vi "课堂.vi"() -> ()   [LabVIEW 2025]
uses:
  <vilib>/Utility/file.llb/Write Delimited Spreadsheet (DBL).vi
  <vilib>/Utility/file.llb/Read Delimited Spreadsheet (DBL).vi
panel:
  out "状态显示 2":string
  out "温度计 2":dbl(slide) scale=0.0..100.0
  out "报警显示 2":bool
  in  "温度下限 2":dbl=10.0
  in  "温度上限 2":dbl=50.0
  out "温度计":dbl(slide) scale=0.0..100.0
  out "报警显示":bool
  out "状态显示":string
  in  "温度下限":dbl=10.0
  in  "温度上限":dbl=50.0
  out "布尔":bool
  in  "滑动杆":dbl(slide) scale=0.0..10.0
  in  "文本 3":string="NIHAO"
  in  "操作(0:open) 3":T1(ring)
  in  "文件路径（使用对话框） 3":path
  in  "数值 3":i32=10
  out "文本 2":string
  in  "操作(0:open) 2":T1(ring)
  in  "文件路径（使用对话框） 2":path
  in  "文本":string
  in  "数值 2":i32=10
  in  "操作(0:open)":T1(ring)
  in  "文件路径（使用对话框）":path
  out "all rows":dbl[][](array[numeric]) caption="所有行"
  in  "number of rows (all:-1)":i32=-1 caption="行数（全部:-1）"
  out "new file path (Not A Path if cancelled) 2":path caption="新建文件路径（取消时为非法路径）"
  in  "file path (dialog if empty) 2":path caption="文件路径（空时为对话框）"
  in  "transpose? (no:F)":bool caption="转置（否:F）"
  in  "format (%.3f)":string="%.3f" caption="格式(%.3f)"
  in  "delimiter (\\t)":string="\t" caption="分隔符(\\t)"
  in  "append to file? (new file:F)":bool caption="添加至文件？（新文件：F）"
  in  "数值":i32=10
  in  "file path (dialog if empty)":path caption="文件路径（空时为对话框）"
  out "new file path (Not A Path if cancelled)":path caption="新建文件路径（取消时为非法路径）"
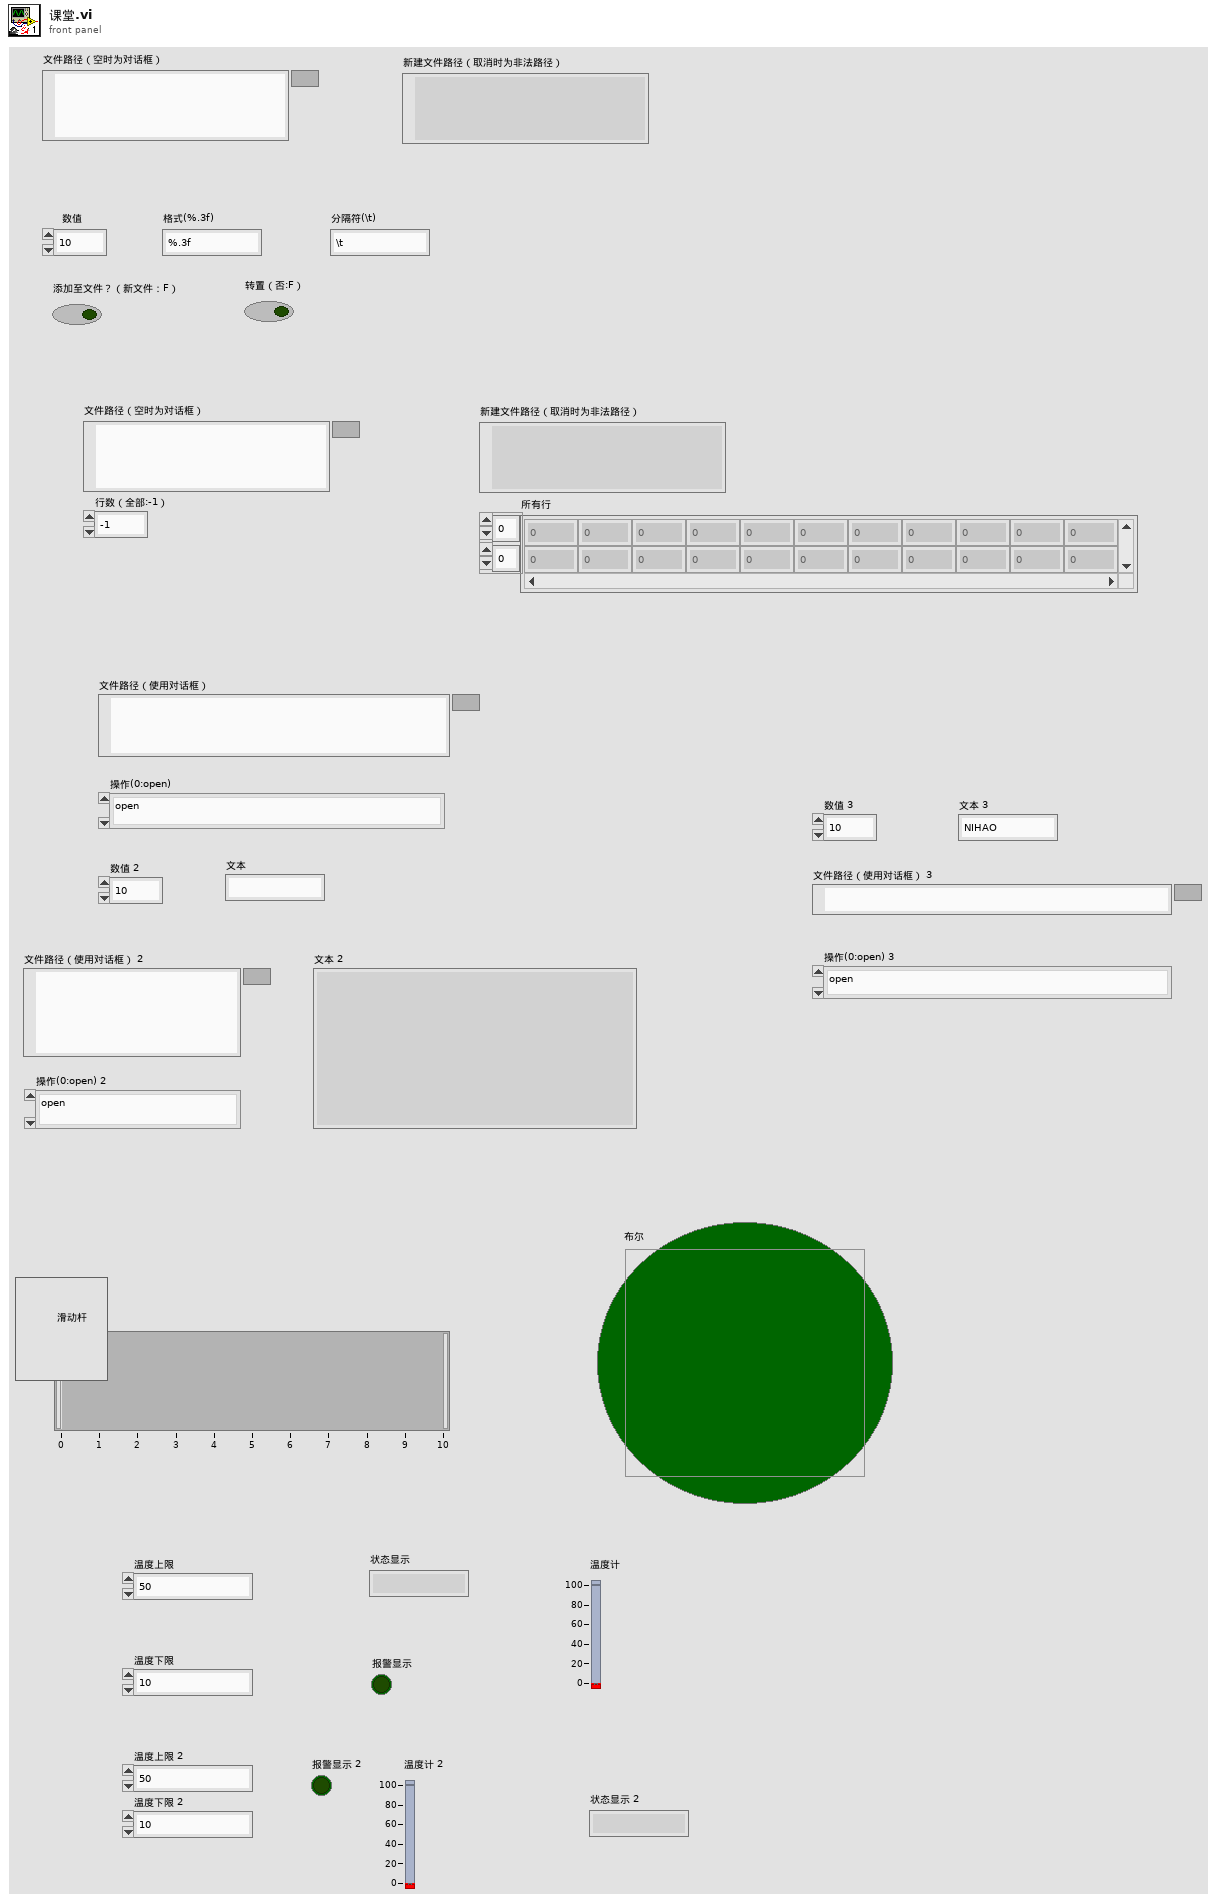
[diagram p1: front panel]
types:
  T1 = enum16{"open", "replace", "create", "open or create", "replace or create", "replace or create with confirmation"}
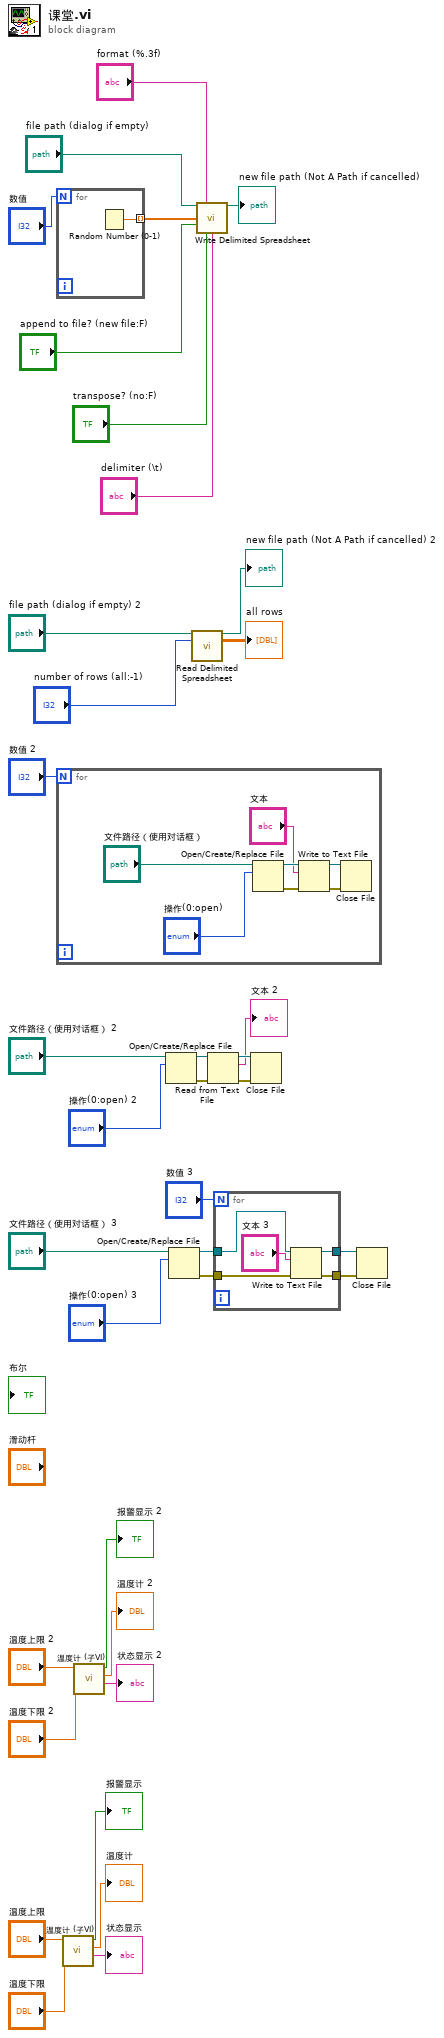
[diagram p0: block diagram]
diagram:
  n1 = for {
    N: "数值" -> [_]
    tunnel: [w38] -> w34 mode=indexing
    n2 = Random Number (0-1)() -> (number: 0 to 1=w38:dbl)
  }
  n3 = for {
    N: "数值 2" -> [_]
    n4 = Open/Create/Replace File(file path (use dialog)="文件路径（使用对话框）", operation (0:open)="操作(0:open)") -> (refnum out=w44:refnum<file>, error out=w40:errorcluster)  [unwired: 4 in, 1 out]
    n5 = Write to Text File(file (use dialog)=w44, text="文本", error in=w40) -> (refnum out=w41:refnum<file>, error out=w39:errorcluster)  [unwired: 1 in, 1 out]
    n6 = Close File(refnum=w41, error in=w39) -> ()  [unwired: 2 out]
  }
  n7 = call "温度计 (子VI).vi"("温度下限"="温度下限", "温度上限"="温度上限") -> ("状态显示"=→"状态显示":string, "温度计"=→"温度计":dbl, "报警显示"=→"报警显示":bool)  [unwired: 7 in]
  n8 = call "温度计 (子VI).vi"("温度下限"="温度下限 2", "温度上限"="温度上限 2") -> ("状态显示"=→"状态显示 2":string, "温度计"=→"温度计 2":dbl, "报警显示"=→"报警显示 2":bool)  [unwired: 7 in]
  n9 = Open/Create/Replace File(file path (use dialog)="文件路径（使用对话框） 2", operation (0:open)="操作(0:open) 2") -> (refnum out=w22:refnum<file>, error out=w19:errorcluster)  [unwired: 4 in, 1 out]
  n10 = Open/Create/Replace File(file path (use dialog)="文件路径（使用对话框） 3", operation (0:open)="操作(0:open) 3") -> (refnum out=w14:refnum<file>, error out=w13:errorcluster)  [unwired: 4 in, 1 out]
  n11 = call-poly <vilib>:"Read Delimited Spreadsheet.vi"("file path (dialog if empty)"="file path (dialog if empty) 2", "number of rows (all:-1)"="number of rows (all:-1)") -> ("new file path (Not A Path if cancelled)"=→"new file path (Not A Path if cancelled) 2":path, "all rows"=→"all rows":dbl[][])  [unwired: 8 in, 4 out]
  n12 = call-poly <vilib>:"Write Delimited Spreadsheet.vi"("file path (dialog if empty)"="file path (dialog if empty)", "format (%.3f)"="format (%.3f)", "1D data"=w34, "append to file? (new file:F)"="append to file? (new file:F)", "transpose? (no:F)"="transpose? (no:F)", "delimiter (\\t)"="delimiter (\\t)") -> ("new file path (Not A Path if cancelled)"=→"new file path (Not A Path if cancelled)":path)  [unwired: 8 in, 1 out]
  n13 = Read from Text File(file (use dialog)=w22, error in=w19) -> (refnum out=w21:refnum<file>, text=→"文本 2":string, error out=w18:errorcluster)  [unwired: 2 in, 1 out]
  n14 = for {
    N: "数值 3" -> [_]
    tunnel: w14 -> [w50]
    tunnel: w13 -> [w48]
    tunnel: [w47] -> w12
    tunnel: [w46] -> w11
    n15 = Write to Text File(file (use dialog)=w50, text="文本 3", error in=w48) -> (refnum out=w46:refnum<file>, error out=w47:errorcluster)  [unwired: 1 in, 1 out]
  }
  n16 = Close File(refnum=w21, error in=w18) -> ()  [unwired: 2 out]
  n17 = Close File(refnum=w11, error in=w12) -> ()  [unwired: 2 out]
